vi "Go to INIT.vi"(8 "error in (no error)":errorcluster, 11 "INIT in":refnum<class "INIT.lvclass">) -> (0 "error out":errorcluster, 3 "State Actor.lvclass":refnum<class "State Actor.lvclass">)   [LabVIEW 2024, in "Chef States.lvlib" / "INIT.lvclass"]
uses:
  INIT.lvclass
  <vilib>/NI/Actors/State Actor/State Actor/State Actor.lvclass
  INIT.lvclass/INIT.ctl
  C:/Users/burakkorkmaz/Desktop/Leveling/repo/Chef States/Chef State/Chef State.lvclass
  C:/Program Files/National Instruments/LabVIEW 2024/vi.lib/NI/Actors/State Actor/State Actor/State Actor.lvclass
  C:/Program Files/National Instruments/LabVIEW 2024/vi.lib/ActorFramework/Actor/Actor.lvclass
  C:/Users/burakkorkmaz/Desktop/Leveling/repo/Chef States/INIT/INIT.lvclass
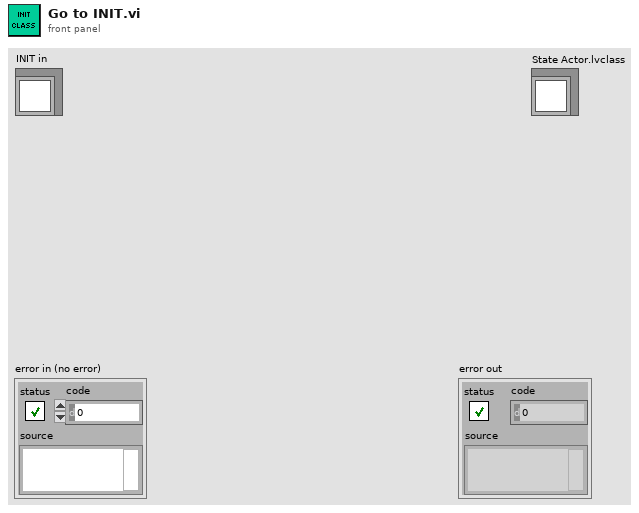
[diagram p1: front panel]
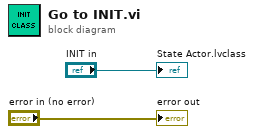
[diagram p0: block diagram]
diagram:
  "error out" <- "error in (no error)"
  "State Actor.lvclass" <- "INIT in"
